vi "PH_AxisGUI_NF.set GUI elements.vi"(0 "i ref in":refnum<vi>, 5 "error in (no error)":errorcluster) -> (14 "i ref out":refnum<vi>, 19 "error out":errorcluster)   [LabVIEW 2014, in "PH_AxisGUI_NF.lvlib"]
uses:
  PH_AxisGUI_NF.lvlib
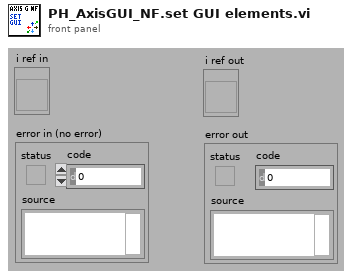
[diagram p1: front panel]
types:
  T1 = typedef "PH_AxisGUI_NF.lvlib/PH_AxisGUI_NF.i attribute.ctl" = cluster{"GUI Refs":cluster{"Delete":refnum<vi>, "Slide 0":refnum<vi>, "Slide 1":refnum<vi>, "Slide 2":refnum<vi>, "Instance Status":refnum<vi>, "Position":refnum<vi>, "Reset":refnum<vi>, "Goal":refnum<vi>, "Go":refnum<vi>}, "Instance":string, "Name Axis 0":string, "Name Axis 1":string, "Name Axis 2":string, "System":string, "Driver Type":T2, "Offset":i32, "Goal":i32}
  T2 = typedef "NF87XX.lvlib/NF87XX.driver Type.ctl" = enum16{"not defined", "3-ch open loop drv", "1-ch closed loop drv"}
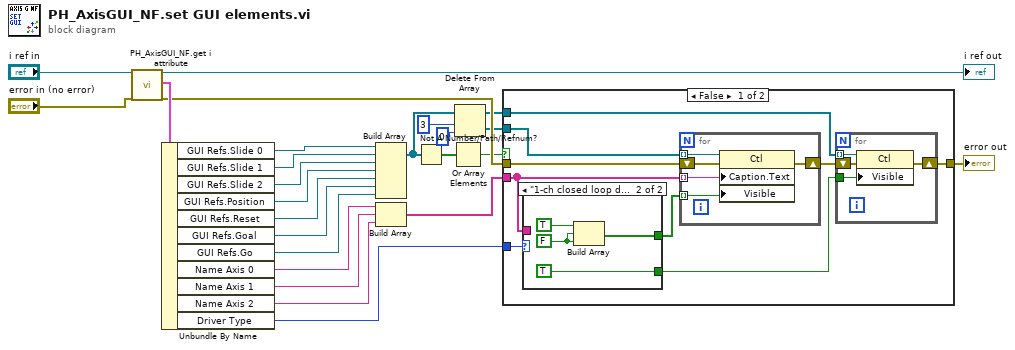
[diagram p0: block diagram]
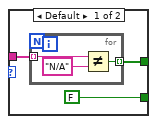
[diagram p2: hidden frame]
diagram:
  n1 = call "PH_AxisGUI_NF.get i attribute.vi"("i ref in"="i ref in", "error in (no error)"="error in (no error)") -> ("i ref out"=→"i ref out":refnum<vi>, "i attribute"=w22:T1, "error out"=w14:errorcluster)  [unwired: 15 in]
  n2 = Unbundle By Name(w22) -> ("GUI Refs.Slide 0"=w21:refnum<vi>, "GUI Refs.Slide 1"=w20:refnum<vi>, "GUI Refs.Slide 2"=w19:refnum<vi>, "GUI Refs.Position"=w9:refnum<vi>, "GUI Refs.Reset"=w8:refnum<vi>, "GUI Refs.Goal"=w7:refnum<vi>, "GUI Refs.Go"=w6:refnum<vi>, "Name Axis 0"=w18:string, "Name Axis 1"=w17:string, "Name Axis 2"=w16:string, "Driver Type"=w11:T2)
  n3 = Build Array(w21, w20, w19, w9, w8, w7, w6) -> (w5:refnum<vi>[])
  n4 = Build Array(w18, w17, w16) -> (w12:string[])
  n5 = Not A Number/Path/Refnum?(number/path/refnum=w5) -> (NaN/Path/Refnum?=w15:bool[])
  n6 = Or Array Elements(Boolean array=w15) -> (logical OR=w10:bool)
  n7 = Delete From Array(array=w5, length=3 ("index"), index=0) -> (deleted portion=w2:refnum<vi>[], array with subset deleted=w1:refnum<vi>[])
  n8 = case shown="False" w10 {
    tunnel: w14 -> [w32 w54]
    tunnel: [w29 w54] -> w13
    tunnel: w12 -> [w31 _]
    tunnel: w11 -> [w34 _]
    tunnel: w2 -> [w27 _]
    tunnel: w1 -> [w26 _]
    frame False {
      n9 = case shown="\"1-ch closed loop drv\"" w34 {
        tunnel: [w46 w51] -> w33
        tunnel: w31 -> [w45 _]
        tunnel: [FALSE TRUE] -> w28
        frame Default {
          n10 = for {
            tunnel: w45 -> [w49] mode=indexing
            tunnel: [w47] -> w46 mode=indexing
            n11 = Not Equal?(x=w49, y="N/A") -> (x != y?=w47:bool)
          }
        }
        frame "1-ch closed loop drv" {
          w52 = FALSE
          n12 = Build Array(TRUE, w52, w52) -> (w51:bool[])
        }
      }
      n13 = for {
        shift-right: [w42] -> w30
        shift-left: w32 -> [w43]
        tunnel: w27 -> [w41] mode=indexing
        tunnel: w31 -> [w40] mode=indexing
        tunnel: w33 -> [w39] mode=indexing
        n14 = property class="Ctl"(reference=w41, error in=w43, "Caption.Text"=w40, "Visible"=w39) -> (error out=w42:errorcluster)  [unwired: 1 out]
      }
      n15 = for {
        shift-right: [w37] -> w29
        shift-left: w30 -> [w38]
        tunnel: w26 -> [w36] mode=indexing
        tunnel: w28 -> [w35]
        n16 = property class="Ctl"(reference=w36, error in=w38, "Visible"=w35) -> (error out=w37:errorcluster)  [unwired: 1 out]
      }
    }
    frame True {
    }
  }
  "error out" <- w13
